vi "Send.vi"(0 "Response Msg in":refnum<class "Response Msg.lvclass">, 1 "Message Priority (Normal)":T2=enum."Normal", 2 "Timeout if waiting(-1ms)":i32=-1, 5 "Actor in":refnum<class "Actor.lvclass">, 7 "Send Function":T1, 9 "Sender (publish)":refnum<class "Sender Msg.lvclass">, 11 "error in (no error)":errorcluster, 12 "Publish Data?(F)":bool) -> (4 "Data":refnum<class "Data.lvclass">, 6 "Actor out":refnum<class "Actor.lvclass">, 8 "Success?":bool, 10 "Waited?":bool, 15 "error out":errorcluster)   [LabVIEW 2020, in "Publisher.lvlib" / "Response Msg.lvclass"]
doc: "Send a Response Msg class. Use the Core Type to specify how to send the message and use Sender to specify a target for the message.\n\nThe Response Msg is similar to the native Reply Msg but the Resoponse Msg supports multiple sending and targetting options and can be setup to be interruptible.\nIf Publish is set to TRUE the Data will sent to and published by the publisher."
uses:
  Response Msg.lvclass
  C:/Current projects/WS/PPL/HDH.Actor Framework.Core.Actor.lvlibp/1abvi3w/vi.lib/ActorFramework/Message/Message.lvclass
  PPL/HDH.Data.Generic.lvlibp/Data.lvclass
  PPL/HDH.Actor Framework.Core.Actor.lvlibp/1abvi3w/vi.lib/ActorFramework/Actor/Actor.lvclass
  Publisher Messages/Sender Msg/Sender Msg.lvclass
  PPL/HDH.Actor Framework.Core.Actor.lvlibp/1abvi3w/vi.lib/ActorFramework/Message Enqueuer/Message Priority.ctl
  Response Core/Controls/Ctl_SendFunction.ctl
  Response Core/Interruptible Reply Core/Interruptible Reply Core.lvclass/Interruptible Reply Core.ctl
  Response Msg.lvclass/Response Msg.ctl
  Response Core/Interruptible Reply Core/Write Timeout.vi
  Response Core/Send and Forget Core/Send and Forget Core.lvclass
  C:/Current projects/WS/HDH.ActorFramework.Core/Actor/Publisher/Messages/Response Msg/Response Core/Response Core/Response Core.lvclass
  Response Core/Request Reply Core/Request Reply Core.lvclass
  Response Core/Interruptible Reply Core/Interruptible Reply Core.lvclass
  Response Core/Response Core/Response Core.lvclass
  PPL/HDH.Actor Framework.Core.Utility.lvlibp
  PPL/HDH.Actor Framework.Core.Actor.lvlibp/1abvi3w/vi.lib/ActorFramework/Message Enqueuer/Message Enqueuer.lvclass
  Publisher.lvlib
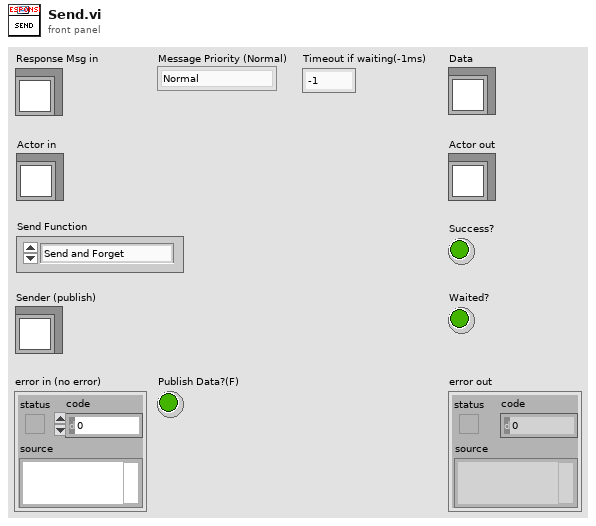
[diagram p1: front panel]
types:
  T1 = typedef "Publisher.lvlib/Ctl_SendFunction.ctl" = enum16{"Send and Forget", "Request Reply", "Await Reply"}
  T2 = typedef "HDH.Actor Framework.Core.Actor.lvlibp/Message Enqueuer.lvclass/Message Priority.ctl" = enum16{"Low", "Normal", "High"}
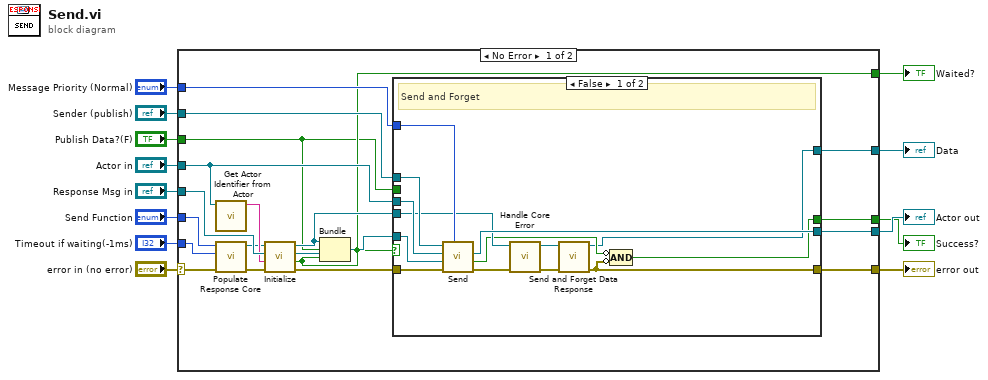
[diagram p0: block diagram]
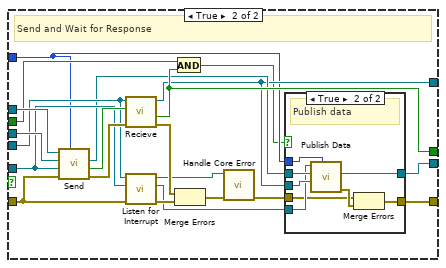
[diagram p2: hidden frame]
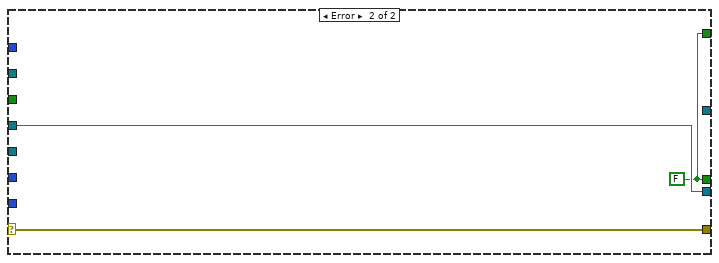
[diagram p4: hidden frame]
diagram:
  n1 = case shown="No Error" "error in (no error)" {
    selector: "error in (no error)" -> [w18 w81]
    tunnel: [w21 w81] -> w12
    tunnel: "Response Msg in" -> [w33 _]
    tunnel: [w28 w80] -> w10
    tunnel: "Actor in" -> [w31 w80]
    tunnel: [w25 w79] -> w8
    tunnel: "Sender (publish)" -> [w32 _]
    tunnel: [w26 _] -> w6
    tunnel: [w20 w79] -> w5
    tunnel: "Message Priority (Normal)" -> [w24 _]
    tunnel: "Publish Data?(F)" -> [w19 _]
    tunnel: "Timeout if waiting(-1ms)" -> [w14 _]
    tunnel: "Send Function" -> [w15 _]
    frame No Error {
      n2 = call "Get Actor Identifier from Actor.vi"("Actor in"=w31) -> ("Actor ID string out"=w30:string)  [unwired: 9 in, 1 out]
      n3 = call "Populate Response Core.vi"("error in (no error)"=w18, "Timeout if waiting(-1ms)"=w14, "Send Function"=w15) -> ("error out"=w17:errorcluster, "Response Core"=w16:refnum<class "Response Core.lvclass">)  [unwired: 7 in]
      n4 = call-dynamic "Initialize.vi"("error in (no error)"=w17, "Enqueuer ID string"=w30, "Response Msg in"=w33, "Response Core in"=w16) -> ("error out"=w27:errorcluster, "Wait for Response?"=w20:bool, "Response Msg out"=w29:refnum<class "Response Msg.lvclass">, "Response Core out"=w22:refnum<class "Response Core.lvclass">)  [unwired: 4 in]
      n5 = Bundle(cluster=w29, w22, w19, w20) -> (w23:refnum<class "Response Msg.lvclass">)
      n6 = case shown="False" w20 {
        tunnel: w32 -> [w46 w68]
        tunnel: w31 -> [w45 w67]
        tunnel: [w44 w53] -> w28
        tunnel: w27 -> [w41 w66]
        tunnel: [w36 w51] -> w26
        tunnel: [w38 w55] -> w25
        tunnel: w24 -> [w47 w49]
        tunnel: w23 -> [w43 w60]
        tunnel: w22 -> [w42 w59]
        tunnel: [w34 w56] -> w21
        tunnel: w19 -> [_ w54]
        frame False {
          # "Send and Forget"
          n7 = call-dynamic "Send.vi"("Message Priority (Normal)"=w47, "error in (no error)"=w41, "Message"=w43, "Actor in"=w45, "Sender Msg in"=w46) -> ("error out"=w40:errorcluster, "Dropped?"=w39:bool, "Actor out"=w44:refnum<class "Actor.lvclass">)  [unwired: 4 in]
          n8 = call-dynamic "Handle Core Error.vi"("error in (no error)"=w40, "Response Core in"=w42) -> ("error out"=w35:errorcluster, "Response Core out"=w37:refnum<class "Response Core.lvclass">)  [unwired: 8 in]
          n9 = call-dynamic "Send and Forget Data Response.vi"("error in (no error)"=w35, "Response Core in"=w37) -> ("error out"=w34:errorcluster, "Data"=w36:refnum<class "Data.lvclass">)  [unwired: 8 in]
          n10 = Compound Arithmetic op=AND(invert w39, invert w34) -> (w38:bool)
        }
        frame True {
          # "Send and Wait for Response"
          n11 = call-dynamic "Send.vi"("Message Priority (Normal)"=w49, "error in (no error)"=w66, "Message"=w60, "Actor in"=w67, "Sender Msg in"=w68) -> ("error out"=w65:errorcluster, "Dropped?"=w64:bool, "Actor out"=w52:refnum<class "Actor.lvclass">)  [unwired: 4 in]
          n12 = call-dynamic "Recieve.vi"("error in (no error)"=w65, "Dropped?"=w64, "Response Core in"=w59) -> ("error out"=w63:errorcluster, "Success?"=w55:bool, "Data"=w51:refnum<class "Data.lvclass">)  [unwired: 6 in]
          n13 = call-dynamic "Listen for Interrupt.vi"("error in (no error)"=w66, "Response Msg in"=w60, "Response Core in"=w59) -> ("error out"=w62:errorcluster, "Response Msg out"=w50:refnum<class "Response Msg.lvclass">, "Response Core out"=w58:refnum<class "Response Core.lvclass">)  [unwired: 6 in]
          n14 = And(x=w54, y=w55) -> (x .and. y?=w48:bool)
          n15 = Merge Errors(w63, w62) -> (w61:errorcluster)
          n16 = call-dynamic "Handle Core Error.vi"("error in (no error)"=w61, "Response Core in"=w58) -> ("error out"=w57:errorcluster)  [unwired: 8 in, 1 out]
          n17 = case shown="True" w48 {
            tunnel: w57 -> [w70 w71]
            tunnel: [w70 w72] -> w56
            tunnel: [w69 w77] -> w53
            tunnel: w52 -> [w69 w76]
            tunnel: w51 -> [_ w75]
            tunnel: w50 -> [_ w74]
            tunnel: w49 -> [_ w73]
            frame False {
              # "Do not publish here"
            }
            frame True {
              # "Publish data"
              n18 = call-dynamic "Publish Data.vi"("Message Priority (Normal)"=w73, "Data"=w75, "Actor in"=w76, "Response Msg"=w74) -> ("error out"=w78:errorcluster, "Actor out"=w77:refnum<class "Actor.lvclass">)  [unwired: 6 in]
              n19 = Merge Errors(w71, w78) -> (w72:errorcluster)
            }
          }
        }
      }
    }
    frame Error {
      w79 = FALSE ("Success?")
    }
  }
  "error out" <- w12
  "Waited?" <- w5
  "Success?" <- w8
  "Data" <- w6
  "Actor out" <- w10
